vi "FTW-Ether-Connections-Query.vi"(0 "Connection":string, 11 "error in":errorcluster) -> (6 "Fetched Address":string, 15 "error out":errorcluster)   [LabVIEW 2015, in "FTW-Ether.lvclass"]
uses:
  FTW-Ether.lvclass
  FTW-Ether-Connections-Action.ctl
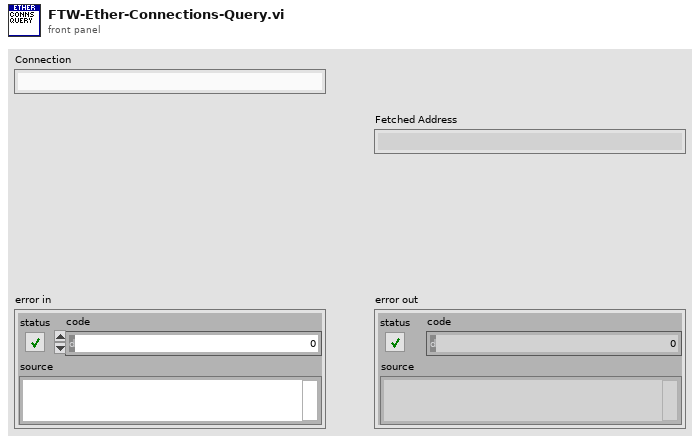
[diagram p1: front panel]
types:
  T1 = typedef "FTW-Ether.lvclass/FTW-Ether-Connections-Action.ctl" = enum8{"Query", "Add", "Reset"}
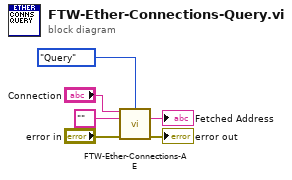
[diagram p0: block diagram]
diagram:
  n1 = call "FTW-Ether-Connections-AE.vi"("Connection"="Connection", "Action"=FTW-Ether-Connections-Action."Query", "Address"="" ("empty string"), "error in"="error in") -> ("Fetched Address"=→"Fetched Address":string, "error out"=→"error out":errorcluster)  [unwired: 10 in]
